vi "FitsCreateFile.vi"(8 "error in (no error)":errorcluster, 10 "Path":path=path "!/home/shrc/HRCSoft/modules/FITS/test/fits_test.fits", 11 "CFitsIO in":refnum<class "CFitsIO.lvclass">) -> (0 "error out":errorcluster, 1 "result":i32, 2 "fd":u64, 3 "CFitsIO out":refnum<class "CFitsIO.lvclass">)   [LabVIEW 2016, in "CFitsIO.lvclass"]
uses:
  CFitsIO.lvclass
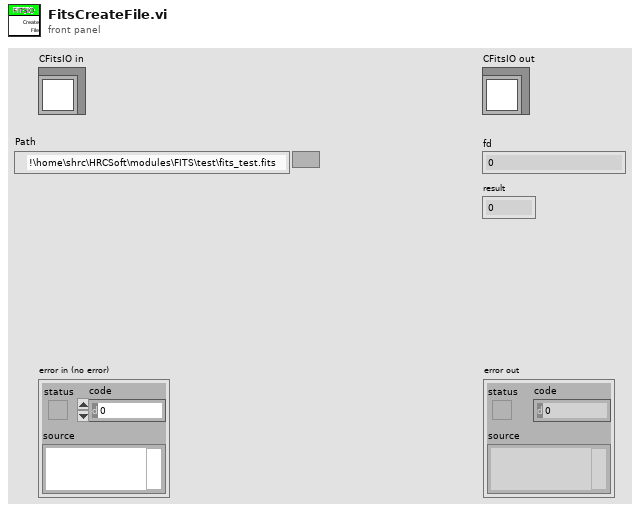
[diagram p1: front panel]
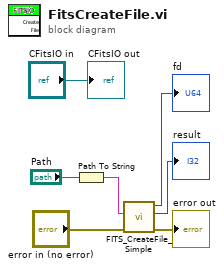
[diagram p0: block diagram]
diagram:
  n1 = Path To String(path="Path") -> (string=w4:string)
  n2 = call "FITS_CreateFile_Simple.vi"("error in"="error in (no error)", "filename"=w4) -> ("error out"=→"error out":errorcluster, "result"=→"result":i32, "fd"=→"fd":u64)  [unwired: 7 out]
  "CFitsIO out" <- "CFitsIO in"
